vi "Patch.vi"(7 "PutRequest":string, 8 "error in (no error)":errorcluster, 9 "Parameter":string, 10 "Request":string, 11 "ByteGSWebAPI-V0 in":refnum<class "ByteGSWebAPI-V0.lvclass">) -> (0 "error out":errorcluster, 3 "ByteGSWebAPI-V0 out":refnum<class "ByteGSWebAPI-V0.lvclass">, 4 "body":string, 6 "headers":string)   [LabVIEW 2019]
uses:
  <vilib>/httpClient/LabVIEWHTTPClient.lvlib
  <vilib>/httpClient/PUTBuffer.vi
  ByteGSWebAPI-V0.lvclass
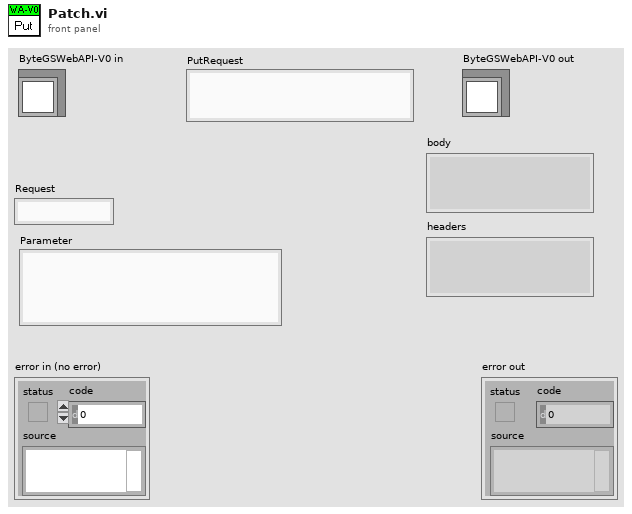
[diagram p1: front panel]
types:
  T1 = typedef "LabVIEWHTTPClient.lvlib/ClientHandle.ctl" = refnum<k1>
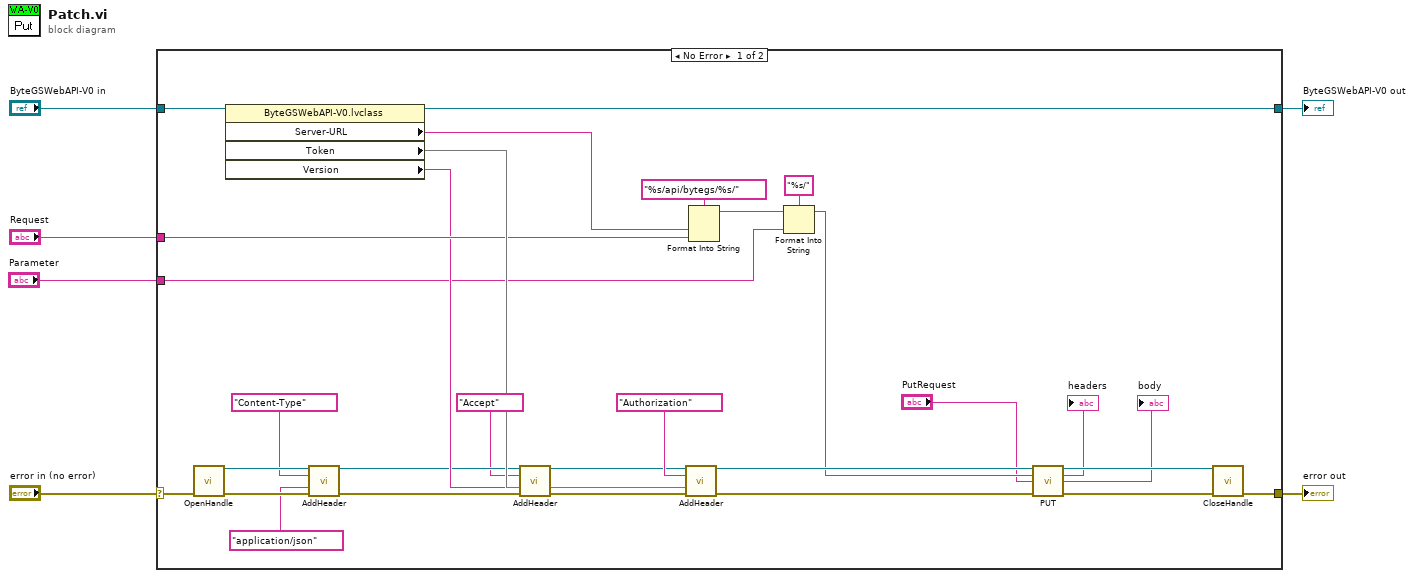
[diagram p0: block diagram]
diagram:
  n1 = case shown="No Error" "error in (no error)" {
    selector: "error in (no error)" -> [w31 w38]
    tunnel: [w30 w38] -> w5
    tunnel: [w29 w37] -> w3
    tunnel: "ByteGSWebAPI-V0 in" -> [w28 w37]
    tunnel: "Request" -> [w24 _]
    tunnel: "Parameter" -> [w10 _]
    frame No Error {
      n2 = call <vilib>:"OpenHandle.vi"("error in (no error)"=w31) -> ("client handle out"=w34:T1, "error out"=w35:errorcluster)  [unwired: 13 in]
      n3 = property class="ByteGSWebAPI-V0.lvclass"(reference=w28) -> (reference out=w29:refnum<class "ByteGSWebAPI-V0.lvclass">, "Server-URL"=w25:string, "Token"=w27, "Version"=w23:string)  [unwired: 1 in, 1 out]
      n4 = call <vilib>:"AddHeader.vi"("client handle"=w34, "header"="Content-Type", "value"="application/json", "error in (no error)"=w35) -> ("client handle out"=w22:T1, "error out"=w21:errorcluster)  [unwired: 10 in]
      n5 = call <vilib>:"AddHeader.vi"("client handle"=w22, "header"="Accept", "value"=w23, "error in (no error)"=w21) -> ("client handle out"=w19:T1, "error out"=w20:errorcluster)  [unwired: 10 in]
      n6 = call <vilib>:"AddHeader.vi"("client handle"=w19, "header"="Authorization", "value"=w27, "error in (no error)"=w20) -> ("client handle out"=w17:T1, "error out"=w16:errorcluster)  [unwired: 10 in]
      n7 = Format Into String(format string="%s/api/bytegs/%s/" ("url"), w25, w24) -> (resulting string=w13:string)  [unwired: 2 in, 1 out]
      n8 = Format Into String(format string="%s/" ("url"), initial string=w13, w10) -> (resulting string=w12:string)  [unwired: 1 in, 1 out]
      n9 = call-poly <vilib>:"PUT.vi"("client handle"=w17, "url"=w12, "buffer"="PutRequest", "error in (no error)"=w16) -> ("client handle out"=w14:T1, "headers"=→"headers":string, "body"=→"body":string, "error out"=w15:errorcluster)  [unwired: 8 in]
      n10 = call <vilib>:"CloseHandle.vi"("client handle"=w14, "error in (no error)"=w15) -> ("error out"=w30:errorcluster)  [unwired: 13 in]
    }
    frame Error {
    }
  }
  "error out" <- w5
  "ByteGSWebAPI-V0 out" <- w3
